vi "Extract hostname.vi"(6 "error in (no error)":errorcluster, 9 "address or URI":string) -> (0 "error out":errorcluster, 3 "hostname":string)   [LabVIEW 2020, in "NI_WFCN.lvlib"]
doc: "If supplied address is a URL, returns its hostname part. Otherwise, return the address unmodified."
uses:
  <vilib>/net/WFCN/NI_WFCN.lvlib
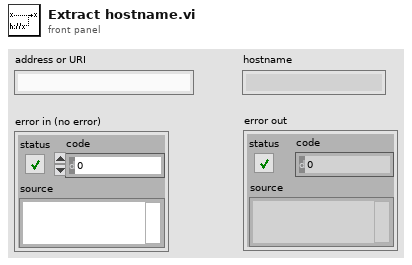
[diagram p1: front panel]
types:
  T1 = typedef "NI_WFCN.lvlib/URIv1.ctl" = cluster{"suffixed scheme":string, "suffixed user":string, "hostname":string, "prefixed port":string, "path":T2, "prefixed query":string, "prefixed fragment":string, "undecoded":T3}
  T2 = typedef "NI_WFCN.lvlib/URI Path Components v1.ctl" = cluster{"elements":string[], "relative":bool}
  T3 = typedef "NI_WFCN.lvlib/URI Undecoded Components v1.ctl" = cluster{"path":string, "authority":string}
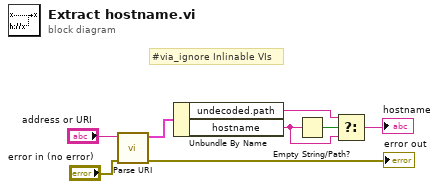
[diagram p0: block diagram]
diagram:
  # "#via_ignore Inlinable VIs"
  n1 = call <vilib>:"Parse URI.vi"("error in (no error)"="error in (no error)", "URI"="address or URI") -> ("error out"=→"error out":errorcluster, "parsed URI"=w7:T1)  [unwired: 8 in]
  n2 = Unbundle By Name(w7) -> ("undecoded.path"=w3:string, "hostname"=w2:string)
  n3 = Empty String/Path?(string/path=w2) -> (empty?=w4:bool)
  n4 = Select(t=w3, s=w4, f=w2) -> (s? t:f=→"hostname":string)
